vi "workspace_cache.set.vi"(8 "error in":errorcluster, 10 "Available Workspaces":refnum<class "workspace.lvclass">[](array[class]), 11 "Nominal Client in":refnum<class "Nominal Client.lvclass">) -> (0 "error out":errorcluster, 3 "Nominal Client out":refnum<class "Nominal Client.lvclass">)   [LabVIEW 2020, in "Nominal Client.lvclass"]
uses:
  Nominal Client.lvclass
  Nominal Client.lvclass/Nominal Client.ctl
  nominal types/workspace/workspace.lvclass
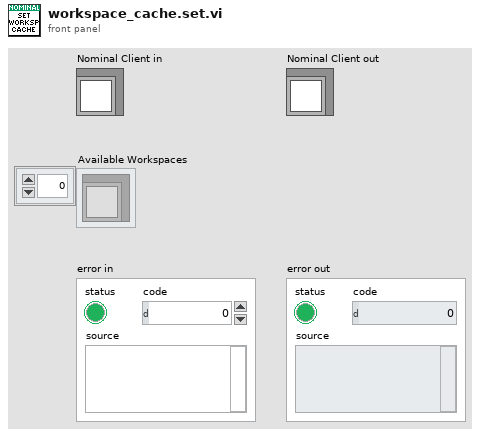
[diagram p1: front panel]
types:
  T1 = typedef "Nominal Client.lvclass/private_data.ctl" = cluster{"API Token":string, "REST Client":refnum<class "REST Client.lvclass">, "workspace":refnum<class "workspace.lvclass">, "Available Workspaces":refnum<class "workspace.lvclass">[]}
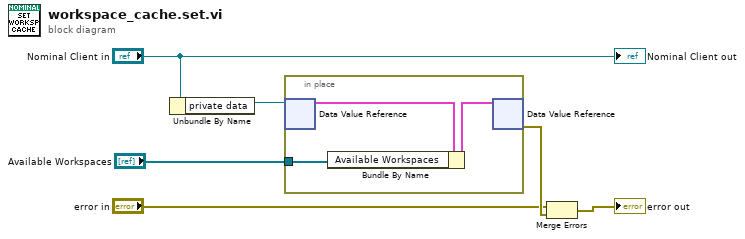
[diagram p0: block diagram]
diagram:
  n1 = Unbundle By Name("Nominal Client in") -> ("private data"=w5:refnum<data-value>)
  n2 = in-place {
    in-place-border: "Available Workspaces" -> [w8]
    n3 = in-place-dvr #1(w5) -> (w9:T1)  [unwired: 1 out]
    n4 = Bundle By Name(cluster=w9, "Available Workspaces"=w8) -> (w7:T1)
    n5 = in-place-dvr #1(w7) -> (w3:errorcluster)  [unwired: 1 out]
  }
  n6 = Merge Errors("error in", w3) -> (→"error out":errorcluster)
  "Nominal Client out" <- "Nominal Client in"
